vi "ListDependencies.vi"(8 "error in (no error)":errorcluster, 11 "SMO in":refnum<class "SMO.lvclass">) -> (0 "error out":errorcluster, 1 "Level":string[](array[string]), 2 "[Dependencies]":refnum<class "SMO.lvclass">[](array[class]), 3 "SMO out":refnum<class "SMO.lvclass">)   [LabVIEW 2013, in "SMO.lvclass"]
uses:
  SMO.lvclass
  SMO.lvclass/SMO.ctl
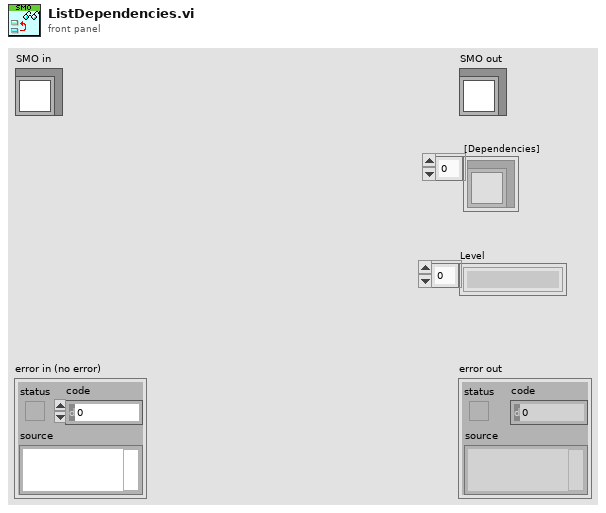
[diagram p1: front panel]
types:
  T1 = typedef "SMO.lvclass/PrivateData--Ref.ctl" = refnum<data-value>
  T2 = typedef "SMO.lvclass/PrivateData--Cluster.ctl" = cluster{"Parent Call":T3, "Registered Processes":T4[], "Sync Notifier":refnum<notifier>, "Process Error Notifier":refnum<notifier>, "Protected Events":T5, "Public Events":T6, "SMO State":T7, "[Dependencies]":T8[], "[Attributes]":refnum<class "Attribute.lvclass">[], "Launcher Close":refnum<notifier>, "Caller Watchdog":refnum<queue>}
  T3 = typedef "SMO.lvclass/Parent Call--Enum.ctl" = enum16{"Allows parent to run", "Does not request parent to run"}
  T4 = typedef "SMO.lvclass/RegisteredProcessData--Cluster.ctl" = cluster{"Name":string, "Static VI Ref":refnum<vi>, "Running":bool, "NotifierRef":u32}
  T5 = typedef "SMO.lvclass/Protected Events.ctl" = cluster{"StopProcesses":refnum<user-event>, "AbortProcesses":refnum<user-event>, "Config Changed":refnum<user-event>, "Dependency":refnum<user-event>}
  T6 = typedef "SMO.lvclass/Public Events.ctl" = cluster{"Error":refnum<user-event>, "State":refnum<user-event>}
  T7 = typedef "SMO.lvclass/SMOState --Enum.ctl" = enum16{"unknown", "Created", "Started", "Stopped"}
  T8 = typedef "SMO.lvclass/SMO Dependency--Cluster.ctl" = cluster{"Dependency":refnum<class "SMO.lvclass">, "Level":string}
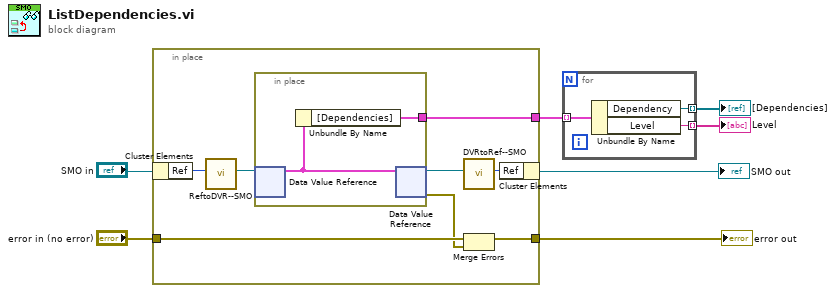
[diagram p0: block diagram]
diagram:
  n1 = in-place {
    in-place-border: "error in (no error)" -> [w11]
    in-place-border: [w9] -> w4
    in-place-border: [w8] -> w3
    n2 = in-place-cluster #1("SMO in") -> ("Ref"=w15:u32)
    n3 = call "ReftoDVR--SMO.vi"("Ref"=w15) -> ("Ref"=w14:T1)  [unwired: 10 in]
    n4 = in-place {
      in-place-border: [w16] -> w8
      n5 = in-place-dvr #2(w14) -> (w17:T2)  [unwired: 1 out]
      n6 = Unbundle By Name(w17) -> ("[Dependencies]"=w16:T8[])
      n7 = in-place-dvr #2(w17) -> (w13:T1, w10:errorcluster)
    }
    n8 = call "DVRtoRef--SMO.vi"("Ref"=w13) -> ("Ref"=w12:u32)  [unwired: 10 in]
    n9 = Merge Errors(w11, w10) -> (w9:errorcluster)
    n10 = in-place-cluster #1("Ref"=w12) -> (→"SMO out":refnum<class "SMO.lvclass">)
  }
  "error out" <- w4
  n11 = for {
    tunnel: w3 -> [w20] mode=indexing
    tunnel: [w19] -> w2 mode=indexing
    tunnel: [w18] -> w1 mode=indexing
    n12 = Unbundle By Name(w20) -> ("Dependency"=w19:refnum<class "SMO.lvclass">, "Level"=w18:string)
  }
  "[Dependencies]" <- w2
  "Level" <- w1
